vi "NF WF1973_74 Initialize.vi"(2 "Error In":errorcluster, 3 "Reset(T)":bool=TRUE, 4 "ID Check(T)":bool=TRUE, 5 "VISAsession":refnum<visa-resource-name>) -> (0 "Error Out":errorcluster, 1 "CopyVISAsession":refnum<visa-resource-name>)   [LabVIEW 2010]
panel:
  # "Yes\nNo"
  # "Yes\nNo"
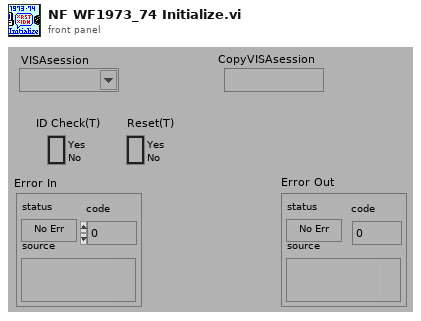
[diagram p1: front panel]
types:
  T1 = cluster{"status":bool, "code":i32, "VI Name":string}
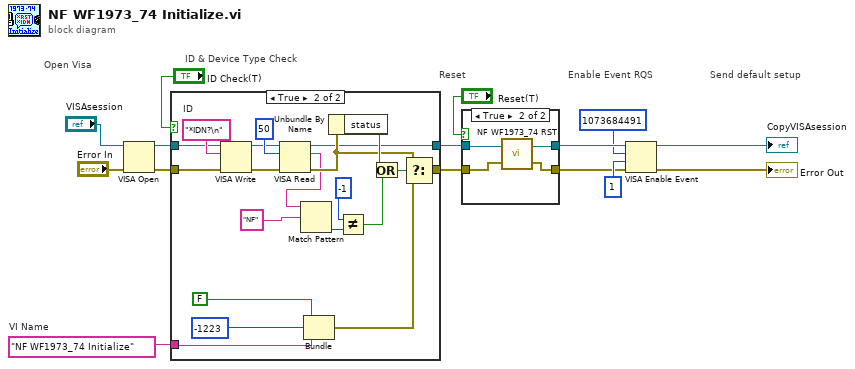
[diagram p0: block diagram]
diagram:
  w6 = "NF WF1973_74 Initialize"  # VI Name
  # "Enable Event RQS"
  # "Send default setup"
  # "ID & Device Type Check"
  # "Reset"
  # "Open Visa"
  n1 = VISA Open(error in (no error)="Error In", VISA resource name="VISAsession") -> (VISA resource name=w12:refnum<visa-resource-name>, error out=w11:errorcluster)  [unwired: 3 in]
  n2 = case shown="TRUE" "ID Check(T)" {
    tunnel: w6 -> [_ w33]
    tunnel: w12 -> [w17 w23]
    tunnel: w11 -> [w16 w26]
    tunnel: [w17 w21] -> w5
    tunnel: [w16 w35] -> w3
    frame False {
    }
    frame True {
      w32 = "*IDN?\n"  # ID
      n3 = VISA Write(VISA resource name=w23, write buffer=w32, error in (no error)=w26) -> (VISA resource name out=w22:refnum<visa-resource-name>, error out=w25:errorcluster)  [unwired: 1 out]
      n4 = VISA Read(VISA resource name=w22, byte count=u32 50, error in (no error)=w25) -> (VISA resource name out=w21:refnum<visa-resource-name>, read buffer=w20:string, error out=w24:errorcluster)  [unwired: 1 out]
      n5 = Match Pattern(string=w20, regular expression="NF") -> (offset past match=w30:i32)  [unwired: 1 in, 3 out]
      n6 = Bundle(FALSE, -1223, "VI Name"=w33) -> (w34:cluster{bool, i32, "VI Name":string})  [unwired: 1 in]
      n7 = Unbundle By Name(w24) -> ("status"=w28:bool)
      n8 = Not Equal?(x=-1, y=w30) -> (x != y?=w18:bool)
      n9 = Or(x=w28, y=w18) -> (x .or. y?=w27:bool)
      n10 = Select(t=w24, s=w27, f=w34) -> (s? t:f=w35:T1)
    }
  }
  n11 = case shown="TRUE" "Reset(T)" {
    tunnel: [w38 w42] -> w7
    tunnel: w5 -> [w39 w40]
    tunnel: [w39 w43] -> w10
    tunnel: w3 -> [w38 w41]
    frame False {
    }
    frame True {
      n12 = call <instrlib>:"NF WF1973_74 RST.vi"("Error In"=w41, "VISAsession"=w40) -> ("Error OUT"=w42:errorcluster, "CopyVISAsession"=w43:refnum<visa-resource-name>)
    }
  }
  n13 = VISA Enable Event(8:w7, 9:u16 1, 10:u32 1073684491, 11:w10) -> (0:→"Error Out":errorcluster, 3:→"CopyVISAsession":refnum<visa-resource-name>)
